vi "data_inter_handle.vi"(8 "error in (no error)":errorcluster caption="错误输入（无错误）", 9 "通信状态":refnum<vi>, 10 "发送报文显示":refnum<vi>, 11 "读取报文显示":refnum<vi>) -> (0 "error out":errorcluster caption="错误输出")   [LabVIEW 2016, in "潮位站数据传输.lvlib"]
uses:
  data_inter/data_inter.lvclass
  tcp/TCP.lvclass
  serial/serial.lvclass
  data_inter/data_inter.lvclass/data_inter.ctl
panel:
  out "serial.lvclass":refnum<class "data_inter.lvclass">
  in  "send":string
  in  "发送数据":bool
  out "数据输出":string
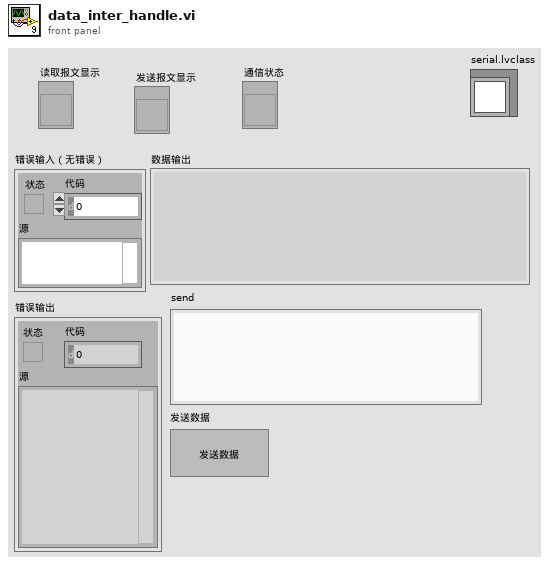
[diagram p1: front panel]
types:
  T1 = cluster{"枚举":enum16{"打开连接", "发送数据", "读取数据", "数据处理", "关闭连接"}, "data":string}
  T2 = cluster{"枚举":enum16{"TCP", "serial"}, "IP":string, "PORT":string, "MN":string, "PW":string, "VISA resource name":refnum<visa-resource-name>, "baud rate":u32}
  T3 = cluster{"IP":string, "PORT":string, "VISA resource name":refnum<visa-resource-name>, "baud rate":u32}
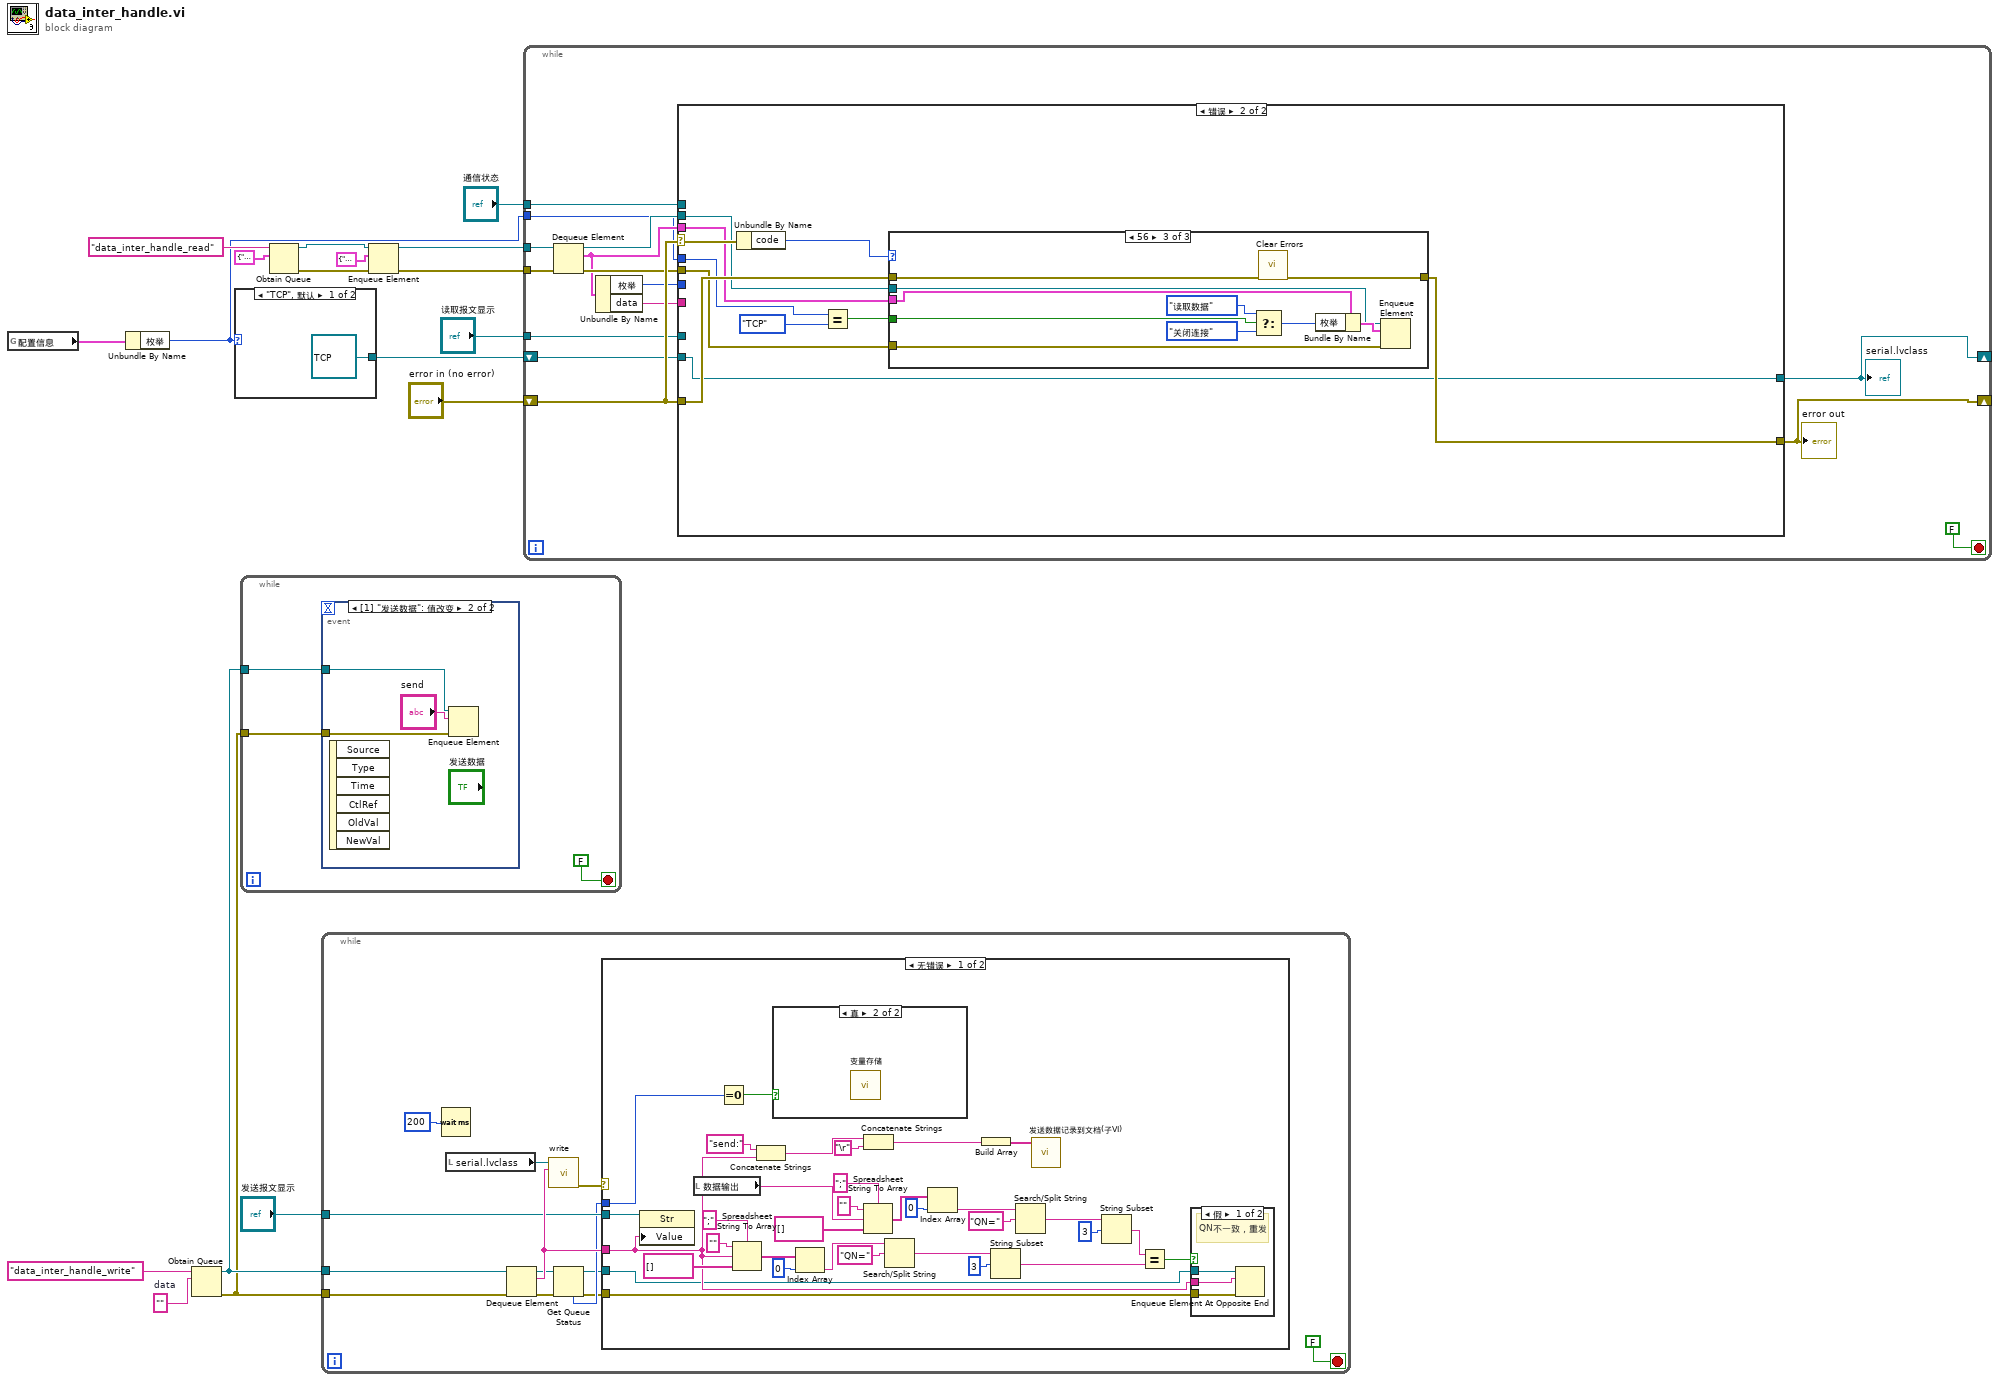
[diagram p0: block diagram]
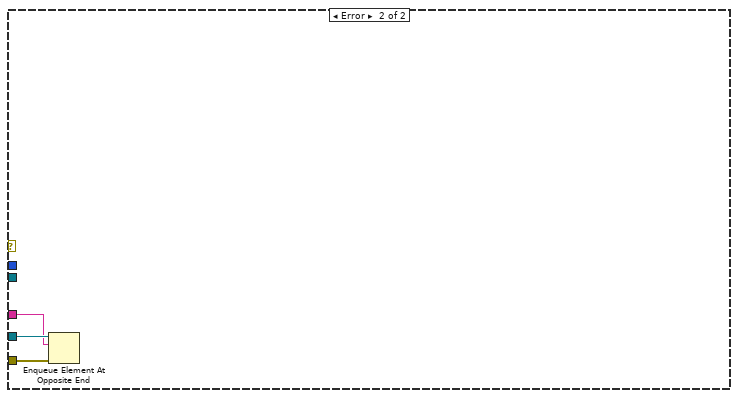
[diagram p4: hidden frame]
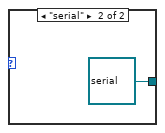
[diagram p5: hidden frame]
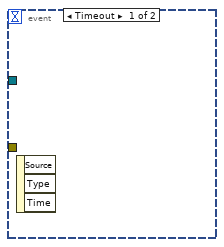
[diagram p6: hidden frame]
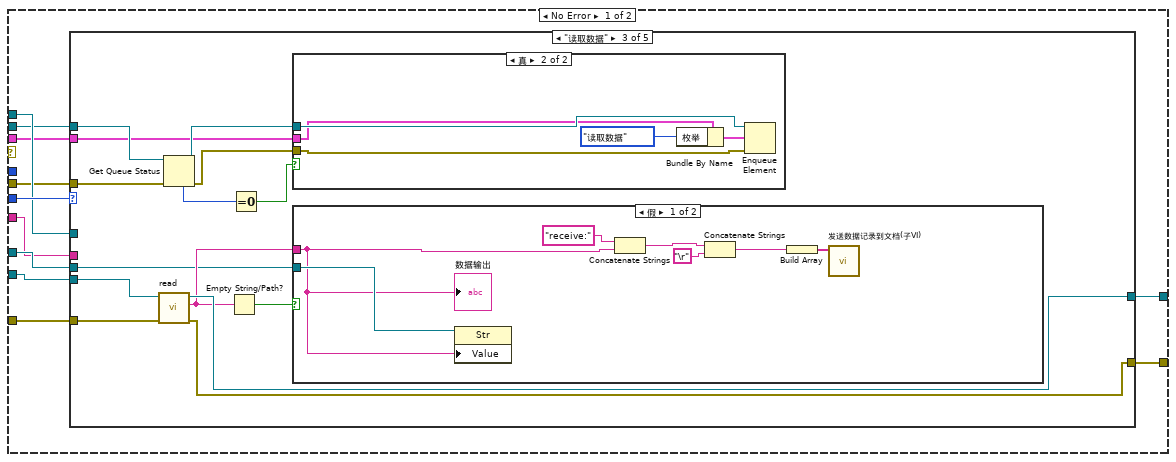
[diagram p7: hidden frame]
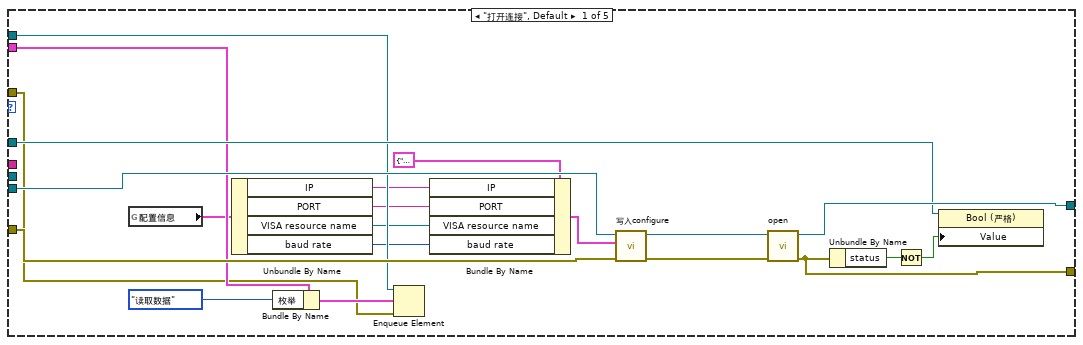
[diagram p8: hidden frame]
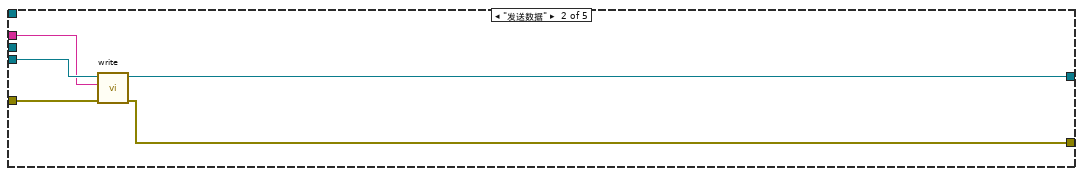
[diagram p9: hidden frame]
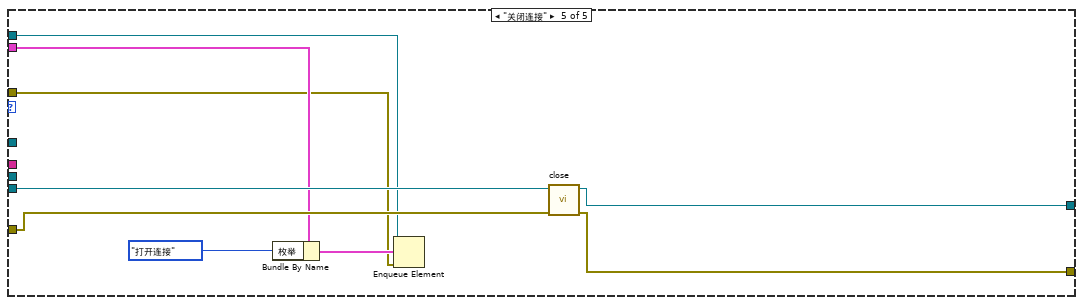
[diagram p13: hidden frame]
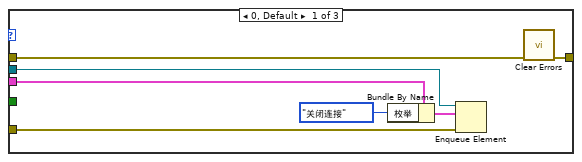
[diagram p14: hidden frame]
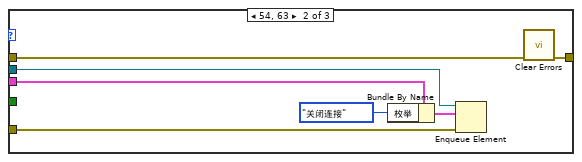
[diagram p15: hidden frame]
diagram:
  w6 = ""  # data
  n1 = global read "断电保存全局.vi" "配置信息"() -> (w2:T2)
  n2 = Unbundle By Name(w2) -> ("枚举"=w1:enum16{"TCP", "serial"})
  n3 = Obtain Queue(name (unnamed)="data_inter_handle_write" ("名称（未命名）"), element data type=w6) -> (queue out=w4:refnum<queue>, error out=w3:errorcluster)  [unwired: 3 in, 1 out]
  n4 = case shown="\"TCP\", 默认" w1 {
    tunnel: [refnum<class "TCP.lvclass"> refnum ("TCP.lvclass") refnum<class "serial.lvclass"> refnum ("serial.lvclass")] -> w18
    frame "TCP", Default {
    }
    frame "serial" {
    }
  }
  n5 = while {
    tunnel: w4 -> [w22]
    tunnel: w3 -> [w21]
    stop <- FALSE stop-if-true
    n6 = event shown="[1] \"发送数据\": 值改变" {
      selector: _ -> [_ _]
      dyn-events: _ -> [_ _]
      timeout: _ -> [_ _]
      tunnel: w22 -> [_ w25]
      tunnel: w21 -> [_ w24]
      event Timeout {
        n7 = event-data() -> ()  [unwired: 1 in, 3 out]
      }
      event "发送数据": Value Change {
        n8 = event-data() -> ()  [unwired: 1 in, 6 out]
        n9 = Enqueue Element(queue=w25, element="send", error in (no error)=w24) -> ()  [unwired: 1 in, 3 out]
      }
    }
  }
  n10 = Obtain Queue(name (unnamed)="data_inter_handle_read" ("名称（未命名）"), element data type=T1 {"枚举"=enum."打开连接", "data"=""}) -> (queue out=w11:refnum<queue>, error out=w10:errorcluster)  [unwired: 3 in, 1 out]
  n11 = while {
    tunnel: w4 -> [w33]
    tunnel: w3 -> [w38]
    tunnel: "发送报文显示" -> [w34]
    stop <- FALSE stop-if-true
    n12 = Wait (ms)(milliseconds to wait=u32 200 ("等待时间（毫秒）")) -> ()  [unwired: 1 out]
    n13 = local read "serial.lvclass"() -> (w39:refnum<class "data_inter.lvclass">)
    n14 = Dequeue Element(queue=w33, error in (no error)=w38) -> (queue out=w32:refnum<queue>, element=w35:string, error out=w31:errorcluster)  [unwired: 1 in, 1 out]
    n15 = call-dynamic "write.vi"("write"=w35, "data_inter 输入"=w39) -> ("error out"=w36:errorcluster)  [unwired: 8 in, 1 out]
    n16 = Get Queue Status(queue=w32, error in (no error)=w31) -> (queue out=w29:refnum<queue>, error out=w28:errorcluster, # elements in queue=w30:i32)  [unwired: 1 in, 5 out]
    n17 = case shown="无错误" w36 {
      tunnel: w29 -> [w41 w78]
      tunnel: w28 -> [w40 w77]
      tunnel: w35 -> [w42 w76]
      tunnel: w34 -> [w67 _]
      tunnel: w30 -> [w66 _]
      frame No Error {
        n18 = property class="Str"(reference=w67, "Value"=w42) -> ()  [unwired: 1 in, 2 out]
        n19 = local read "数据输出"() -> (w43:string)
        n20 = Equal To 0?(x=w66) -> (x = 0?=w65:bool)
        n21 = Spreadsheet String To Array(delimiter (Tab)=";" ("分隔符(Tab)"), format string="" ("格式字符串"), spreadsheet string=w42, array type (2D Dbl)=string[] [] ("数组")) -> (array=w55:string[])
        n22 = Concatenate Strings("send:" ("字符串"), w42) -> (w70:string)
        n23 = case shown="真" w65 {
          frame False {
          }
          frame True {
            n24 = call "变量存储.vi"() -> ()  [unwired: 12 in]
          }
        }
        n25 = Index Array(array=w55, index=0 ("索引")) -> (element=w61:string)
        n26 = Spreadsheet String To Array(delimiter (Tab)=";" ("分隔符(Tab)"), format string="" ("格式字符串"), spreadsheet string=w43, array type (2D Dbl)=string[] [] ("数组")) -> (array=w50:string[])
        n27 = Concatenate Strings(w70, "\r") -> (w68:string)
        n28 = Search/Split String(string=w61, search string/char (-)="QN=" ("搜索字符串/字符(-)")) -> (match + rest of string=w58:string)  [unwired: 1 in, 2 out]
        n29 = Index Array(array=w50, index=0 ("索引")) -> (element=w44:string)
        n30 = Build Array(w68) -> (w72:string[])
        n31 = String Subset(string=w58, offset (0)=3 ("偏移量(0)")) -> (substring=w63:string)  [unwired: 1 in]
        n32 = Search/Split String(string=w44, search string/char (-)="QN=" ("搜索字符串/字符(-)")) -> (match + rest of string=w47:string)  [unwired: 1 in, 2 out]
        n33 = call "发送数据记录到文档(子VI).vi"("数组"=w72) -> ()  [unwired: 9 in, 1 out]
        n34 = String Subset(string=w47, offset (0)=3 ("偏移量(0)")) -> (substring=w62:string)  [unwired: 1 in]
        n35 = Equal?(x=w62, y=w63) -> (x = y?=w64:bool)
        n36 = case shown="假" w64 {
          tunnel: w42 -> [w73 _]
          tunnel: w41 -> [w75 _]
          tunnel: w40 -> [w74 _]
          frame False {
            # "QN不一致，重发"
            n37 = Enqueue Element At Opposite End(queue=w75, element=w73, error in (no error)=w74) -> ()  [unwired: 1 in, 3 out]
          }
          frame True {
            # "QN一致"
          }
        }
      }
      frame Error {
        n38 = Enqueue Element At Opposite End(queue=w78, element=w76, error in (no error)=w77) -> ()  [unwired: 1 in, 3 out]
      }
    }
  }
  n39 = Enqueue Element(queue=w11, element=T1 {"枚举"=enum."打开连接", "data"=""} ("元素"), error in (no error)=w10) -> (queue out=w12:refnum<queue>, error out=w9:errorcluster)  [unwired: 1 in, 1 out]
  n40 = while {
    shift-right: [w88] -> _
    shift-left: "error in (no error)" -> [w92]
    shift-right: [w91] -> _
    shift-left: w18 -> [w90]
    tunnel: "读取报文显示" -> [w89]
    tunnel: "通信状态" -> [w87]
    tunnel: w12 -> [w86]
    tunnel: w9 -> [w85]
    tunnel: w1 -> [w79]
    stop <- FALSE stop-if-true
    n41 = Dequeue Element(queue=w86, error in (no error)=w85) -> (queue out=w82:refnum<queue>, element=w80:T1, error out=w81:errorcluster)  [unwired: 1 in, 1 out]
    n42 = Unbundle By Name(w80) -> ("枚举"=w84:enum16{"打开连接", "发送数据", "读取数据", "数据处理", "关闭连接"}, "data"=w83:string)
    n43 = case shown="错误" w92 {
      selector: w92 -> [_ w178]
      tunnel: w84 -> [w104 _]
      tunnel: w92 -> [w103 w176]
      tunnel: [w102 w175] -> w88
      tunnel: [w101 w174] -> w91
      tunnel: w90 -> [w100 w174]
      tunnel: w89 -> [w99 _]
      tunnel: w87 -> [w98 _]
      tunnel: w83 -> [w97 _]
      tunnel: w82 -> [w96 w173]
      tunnel: w81 -> [w95 w171]
      tunnel: w80 -> [w94 w172]
      tunnel: w79 -> [_ w170]
      frame No Error {
        n44 = case shown="\"读取数据\"" w104 {
          tunnel: w103 -> [w124 w129 w143 w157 w167]
          tunnel: [w116 w127 w142 w157 w164] -> w102
          tunnel: [w122 w128 w141 w158 w165] -> w101
          tunnel: w100 -> [w125 w130 w144 w158 w166]
          tunnel: w99 -> [_ _ w138 _ _]
          tunnel: w98 -> [w115 _ _ _ _]
          tunnel: w97 -> [_ w126 _ _ _]
          tunnel: w96 -> [w112 _ w137 _ w163]
          tunnel: w95 -> [w110 _ w136 _ w159]
          tunnel: w94 -> [w111 _ w131 _ w162]
          frame "打开连接", Default {
            n45 = global read "断电保存全局.vi" "配置信息"() -> (w109:T2)
            n46 = Unbundle By Name(w109) -> ("IP"=w108:string, "PORT"=w107:string, "VISA resource name"=w106:refnum<visa-resource-name>, "baud rate"=w105:u32)
            n47 = Bundle By Name(cluster=w111, "枚举"=enum16{"打开连接", "发送数据", "读取数据", "数据处理", "关闭连接"}."读取数据") -> (w113:T1)
            n48 = Enqueue Element(queue=w112, element=w113, error in (no error)=w110) -> ()  [unwired: 1 in, 3 out]
            n49 = Bundle By Name(cluster=T3 {"IP"="", "PORT"="", "VISA resource name"="", "baud rate"=115200} ("configure"), "IP"=w108, "PORT"=w107, "VISA resource name"=w106, "baud rate"=w105) -> (w120:T3)
            n50 = call "写入configure.vi"("error in (no error)"=w124, "configure"=w120, "data_inter输入"=w125) -> ("error out"=w121:errorcluster, "data_inter输出"=w123:refnum<class "data_inter.lvclass">)  [unwired: 7 in]
            n51 = call-dynamic "open.vi"("error in (no error)"=w121, "data_inter 输入"=w123) -> ("error out"=w116:errorcluster, "data_inter 输出"=w122:refnum<class "data_inter.lvclass">)  [unwired: 8 in]
            n52 = Unbundle By Name(w116) -> ("status"=w118:bool)
            n53 = Not(x=w118) -> (.not. x?=w117:bool)
            n54 = property class="Bool (严格)"(reference=w115, "Value"=w117) -> ()  [unwired: 1 in, 2 out]
          }
          frame "发送数据" {
            n55 = call-dynamic "write.vi"("error in (no error)"=w129, "write"=w126, "data_inter 输入"=w130) -> ("error out"=w127:errorcluster, "data_inter 输出"=w128:refnum<class "data_inter.lvclass">)  [unwired: 7 in]
          }
          frame "读取数据" {
            n56 = call-dynamic "read.vi"("error in (no error)"=w143, "data_inter 输入"=w144) -> ("error out"=w142:errorcluster, "read"=w139:string, "data_inter 输出"=w141:refnum<class "data_inter.lvclass">)  [unwired: 7 in]
            n57 = Get Queue Status(queue=w137, error in (no error)=w136) -> (queue out=w134:refnum<queue>, error out=w133:errorcluster, # elements in queue=w135:i32)  [unwired: 1 in, 5 out]
            n58 = Empty String/Path?(string/path=w139) -> (empty?=w140:bool)
            n59 = Equal To 0?(x=w135) -> (x = 0?=w132:bool)
            n60 = case shown="真" w132 {
              tunnel: w134 -> [_ w149]
              tunnel: w133 -> [_ w148]
              tunnel: w131 -> [_ w147]
              frame False {
              }
              frame True {
                n61 = Bundle By Name(cluster=w147, "枚举"=enum16{"打开连接", "发送数据", "读取数据", "数据处理", "关闭连接"}."读取数据") -> (w145:T1)
                n62 = Enqueue Element(queue=w149, element=w145, error in (no error)=w148) -> ()  [unwired: 1 in, 3 out]
              }
            }
            n63 = case shown="假" w140 {
              tunnel: w139 -> [w150 _]
              tunnel: w138 -> [w151 _]
              frame False {
                n64 = property class="Str"(reference=w151, "Value"=w150) -> ()  [unwired: 1 in, 2 out]
                n65 = Concatenate Strings("receive:" ("字符串"), w150) -> (w154:string)
                n66 = Concatenate Strings(w154, "\r") -> (w152:string)
                n67 = Build Array(w152) -> (w156:string[])
                n68 = call "发送数据记录到文档(子VI).vi"("数组"=w156) -> ()  [unwired: 9 in, 1 out]
                "数据输出" <- w150
              }
              frame True {
              }
            }
          }
          frame "数据处理" {
          }
          frame "关闭连接" {
            n69 = Bundle By Name(cluster=w162, "枚举"=enum16{"打开连接", "发送数据", "读取数据", "数据处理", "关闭连接"}."打开连接") -> (w160:T1)
            n70 = Enqueue Element(queue=w163, element=w160, error in (no error)=w159) -> ()  [unwired: 1 in, 3 out]
            n71 = call-dynamic "close.vi"("error in (no error)"=w167, "data_inter 输入"=w166) -> ("error out"=w164:errorcluster, "data_inter 输出"=w165:refnum<class "data_inter.lvclass">)  [unwired: 8 in]
          }
        }
      }
      frame Error {
        n72 = Unbundle By Name(w178) -> ("code"=w177:i32)
        n73 = Equal?(x=w170, y=enum16{"TCP", "serial"}."TCP") -> (x = y?=w168:bool)
        n74 = case shown="56" w177 {
          tunnel: w176 -> [w185 w191 w201]
          tunnel: [w184 w192 w202] -> w175
          tunnel: w173 -> [w181 w186 w198]
          tunnel: w172 -> [w180 w188 w199]
          tunnel: w171 -> [w179 w187 w197]
          tunnel: w168 -> [_ _ w196]
          frame 0, Default {
            n75 = Bundle By Name(cluster=w180, "枚举"=enum16{"打开连接", "发送数据", "读取数据", "数据处理", "关闭连接"}."关闭连接") -> (w183:T1)
            n76 = Enqueue Element(queue=w181, element=w183, error in (no error)=w179) -> ()  [unwired: 1 in, 3 out]
            n77 = call <vilib>:"Clear Errors.vi"("error in (no error)"=w185) -> ("error out"=w184:errorcluster)  [unwired: 5 in, 1 out]
          }
          frame 54, 63 {
            n78 = Bundle By Name(cluster=w188, "枚举"=enum16{"打开连接", "发送数据", "读取数据", "数据处理", "关闭连接"}."关闭连接") -> (w190:T1)
            n79 = Enqueue Element(queue=w186, element=w190, error in (no error)=w187) -> ()  [unwired: 1 in, 3 out]
            n80 = call <vilib>:"Clear Errors.vi"("error in (no error)"=w191) -> ("error out"=w192:errorcluster)  [unwired: 5 in, 1 out]
          }
          frame 56 {
            n81 = Select(t=enum16{"打开连接", "发送数据", "读取数据", "数据处理", "关闭连接"}."读取数据" ("枚举"), s=w196, f=enum16{"打开连接", "发送数据", "读取数据", "数据处理", "关闭连接"}."关闭连接" ("枚举")) -> (s? t:f=w193:enum16{"打开连接", "发送数据", "读取数据", "数据处理", "关闭连接"})
            n82 = call <vilib>:"Clear Errors.vi"("error in (no error)"=w201) -> ("error out"=w202:errorcluster)  [unwired: 5 in, 1 out]
            n83 = Bundle By Name(cluster=w199, "枚举"=w193) -> (w200:T1)
            n84 = Enqueue Element(queue=w198, element=w200, error in (no error)=w197) -> ()  [unwired: 1 in, 3 out]
          }
        }
      }
    }
    "error out" <- w88
    "serial.lvclass" <- w91
  }
